vi "IT7800 Info.vi"(8 "error in":errorcluster, 11 "VISA in":refnum<visa-resource-name>="TCPIP::192.168.0.252") -> (0 "error out":errorcluster, 2 "IT7800 Info":T1, 3 "VISA out":refnum<visa-resource-name>)   [LabVIEW 2025]
panel:
  # "IP7800 Driver V0.10\nModel information"
  # "06.05.2025"
  # "Andrej Valand"
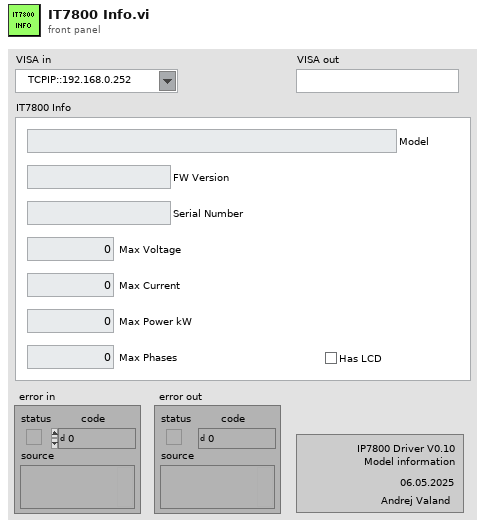
[diagram p1: front panel]
types:
  T1 = cluster{"Model":string, "FW Version":string, "Serial Number":string, "Max Voltage":dbl, "Max Current":dbl, "Max Power kW":dbl, "Max Phases":u8, "Has LCD":bool}
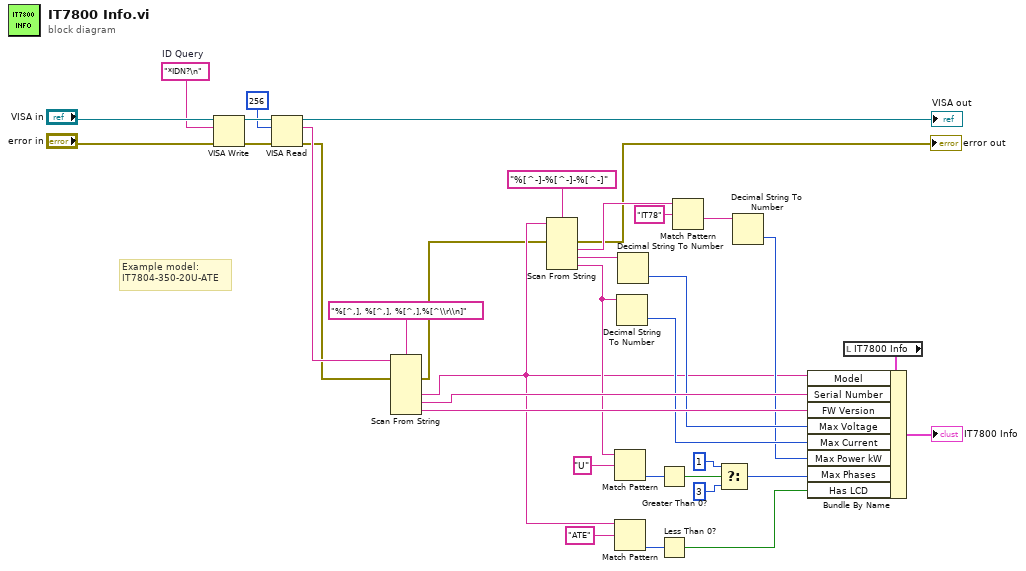
[diagram p0: block diagram]
diagram:
  w28 = "*IDN?\n"  # ID Query
  # "Example model:\nIT7804-350-20U-ATE"
  n1 = VISA Write(VISA resource name="VISA in", write buffer=w28, error in (no error)="error in") -> (VISA resource name out=w35:refnum<visa-resource-name>, error out=w34:errorcluster)  [unwired: 1 out]
  n2 = VISA Read(VISA resource name=w35, byte count=u32 256, error in (no error)=w34) -> (VISA resource name out=→"VISA out":refnum<visa-resource-name>, read buffer=w9:string, error out=w2:errorcluster)  [unwired: 1 out]
  n3 = Scan From String(format string="%[^,], %[^,], %[^,],%[^\\r\\n]", input string=w9, error in=w2) -> (error out=w1:errorcluster, output 2=w4:string, output 3=w26:string, output 4=w25:string)  [unwired: 6 in, 2 out]
  n4 = Scan From String(format string="%[^-]-%[^-]-%[^-]", input string=w4, error in=w1) -> (error out=→"error out":errorcluster, output 1=w19:string, output 2=w22:string, output 3=w8:string)  [unwired: 4 in, 2 out]
  n5 = Match Pattern(string=w8, regular expression="U") -> (offset past match=w14:i32)  [unwired: 1 in, 3 out]
  n6 = Match Pattern(string=w4, regular expression="ATE") -> (offset past match=w6:i32)  [unwired: 1 in, 3 out]
  n7 = Decimal String To Number(string=w8) -> (number=w20:i32)  [unwired: 2 in, 1 out]
  n8 = Decimal String To Number(string=w22) -> (number=w21:i32)  [unwired: 2 in, 1 out]
  n9 = Greater Than 0?(x=w14) -> (x > 0?=w13:bool)
  n10 = Less Than 0?(x=w6) -> (x < 0?=w5:bool)
  n11 = Match Pattern(string=w19, regular expression="IT78") -> (after substring=w17:string)  [unwired: 1 in, 3 out]
  n12 = Select(t=u8 1, s=w13, f=u8 3) -> (s? t:f=w12:u8)
  n13 = Decimal String To Number(string=w17) -> (number=w16:i32)  [unwired: 2 in, 1 out]
  n14 = local read "IT7800 Info"() -> (w27:T1)
  n15 = Bundle By Name(cluster=w27, "Model"=w4, "Serial Number"=w26, "FW Version"=w25, "Max Voltage"=w21, "Max Current"=w20, "Max Power kW"=w16, "Max Phases"=w12, "Has LCD"=w5) -> (→"IT7800 Info":T1)
